vi "Get Monitor Queue Status Section and Channels.vi"(8 "error in":errorcluster, 11 "Custom Device Ref in":T1 format="%.0x") -> (0 "error out":errorcluster, 1 "Monitor Queue Status channel Refs":T1[](array[typedef]) format="%.0x", 2 "Monitor Queue Status Section Ref out":T1 format="%.0x", 3 "Custom Device Ref out":T1 format="%.0x", 4 "Found?":bool)   [LabVIEW 2020, in "afdx_custom_device Scripting.lvlib"]
uses:
  afdx_custom_device Scripting.lvlib
  <vilib>/NI VeriStand/Custom Device API/Custom Device Item Ref.ctl
  Constants.vi
  <vilib>/NI VeriStand/Custom Device Tools/Custom Device Utility Library/NI VeriStand - Search for Item by GUID.vi
  <vilib>/NI VeriStand/Custom Device Tools/Custom Device Utility Library/NI VeriStand - Search for Item by Name.vi
  <vilib>/NI VeriStand/Custom Device Tools/Custom Device Utility Library/Custom Device Utility Library.lvlib
  <vilib>/NI VeriStand/Custom Device API/Custom Device API.lvlib
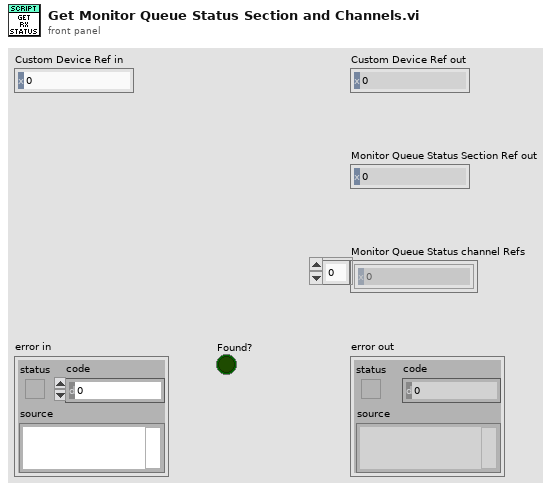
[diagram p1: front panel]
types:
  T1 = typedef "Custom Device API.lvlib/Custom Device Item Ref.ctl" = u64
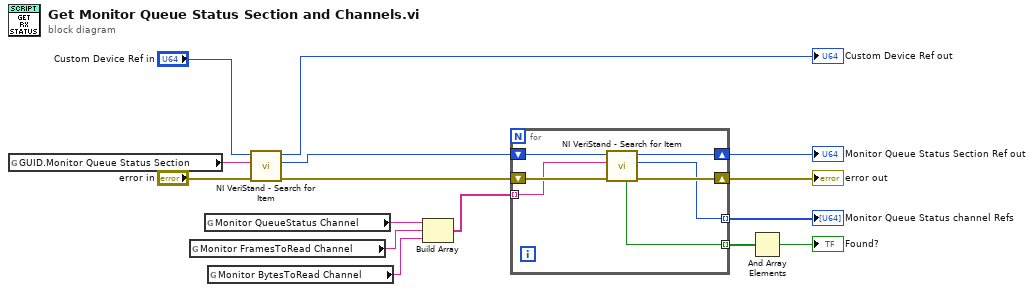
[diagram p0: block diagram]
diagram:
  n1 = global read "Constants.vi" "GUID.Monitor Queue Status Section"() -> (w12:string)
  n2 = global read "Constants.vi" "Monitor FramesToRead Channel"() -> (w5:string)
  n3 = global read "Constants.vi" "Monitor QueueStatus Channel"() -> (w6:string)
  n4 = global read "Constants.vi" "Monitor BytesToRead Channel"() -> (w4:string)
  n5 = call-poly <vilib>:"NI VeriStand - Search for Item.vi"("error in"="error in", "Item GUID"=w12, "Section Ref in"="Custom Device Ref in") -> ("error out"=w13:errorcluster, "Item Ref"=w10:T1, "Section Ref out"=→"Custom Device Ref out":T1)  [unwired: 5 in, 1 out]
  n6 = Build Array(w6, w5, w4) -> (w3:string[])
  n7 = for {
    tunnel: [w18] -> w7 mode=indexing
    shift-right: [w19] -> w8
    shift-left: w13 -> [w22]
    tunnel: w3 -> [w17] mode=indexing
    shift-right: [w21] -> w11
    shift-left: w10 -> [w20]
    tunnel: [w16] -> w2 mode=indexing
    n8 = call-poly <vilib>:"NI VeriStand - Search for Item.vi"("error in"=w22, "Item Name"=w17, "Section Ref in"=w20) -> ("error out"=w19:errorcluster, "Item Ref"=w18:T1, "Section Ref out"=w21:T1, "Found"=w16:bool)  [unwired: 5 in]
  }
  "Monitor Queue Status Section Ref out" <- w11
  "error out" <- w8
  "Monitor Queue Status channel Refs" <- w7
  n9 = And Array Elements(Boolean array=w2) -> (logical AND=→"Found?":bool)
